vi "GPR Init.vi"(3 "Container State":T10, 4 "Previous State":variant, 5 "Previous Version":T9) -> (2 "Current State":T1={"GPR Graph Info"={"Display Type"=enum."Intensity Plot", "Display Info"={"X Scale"={"X Scale Label"=TRUE, "X Scale Name"="Trace #", "X Scale Visible"=TRUE, "dx"=1.0}, "Y Scale"={"X Scale Label"=TRUE, "X Scale Name"="Time (s)", "X Scale Visible"=TRUE, "dt"=4e-10}, "BackGround Color"=16448250}, "Trace Options"={"Trace Amplitude"=1.0, "Trace Color"=0, "Fill options"=enum."No Fill"}, "Intensity Options"={"Color Scale"=enum."RWB"}}, "Transpose Data"=FALSE, "Run-time Edit"=FALSE, "Clear Request"=FALSE})   [LabVIEW 2009, in "GPR.xctl"]
uses:
  GPR.xctl
  GPR State.ctl
  Controls/GPR Graph Info.ctl
  Controls/Display Types.ctl
  Controls/Display Info.ctl
  Controls/Trace Options.ctl
  Controls/Fill Options.ctl
  Controls/Intensity Options.ctl
  Controls/Color Scales.ctl
  <vilib>/_xctls/Container State.ctl
  <vilib>/_xctls/Version.ctl
  <vilib>/_xctls/XControlSupport.lvlib
panel:
  in  "Default Indicator State":T1={"GPR Graph Info"={"Display Type"=enum."Intensity Plot", "Display Info"={"X Scale"={"X Scale Label"=TRUE, "X Scale Name"="Trace #", "X Scale Visible"=TRUE, "dx"=1.0}, "Y Scale"={"X Scale Label"=TRUE, "X Scale Name"="Time (s)", "X Scale Visible"=TRUE, "dt"=4e-10}, "BackGround Color"=16448250}, "Trace Options"={"Trace Amplitude"=1.0, "Trace Color"=0, "Fill options"=enum."No Fill"}, "Intensity Options"={"Color Scale"=enum."RWB"}}, "Transpose Data"=FALSE, "Run-time Edit"=FALSE, "Clear Request"=FALSE}
  in  "Default Control State":T1={"GPR Graph Info"={"Display Type"=enum."Intensity Plot", "Display Info"={"X Scale"={"X Scale Label"=TRUE, "X Scale Name"="Trace #", "X Scale Visible"=TRUE, "dx"=1.0}, "Y Scale"={"X Scale Label"=TRUE, "X Scale Name"="Time (s)", "X Scale Visible"=TRUE, "dt"=4e-10}, "BackGround Color"=16448250}, "Trace Options"={"Trace Amplitude"=1.0, "Trace Color"=0, "Fill options"=enum."No Fill"}, "Intensity Options"={"Color Scale"=enum."RWB"}}, "Transpose Data"=FALSE, "Run-time Edit"=FALSE, "Clear Request"=FALSE}
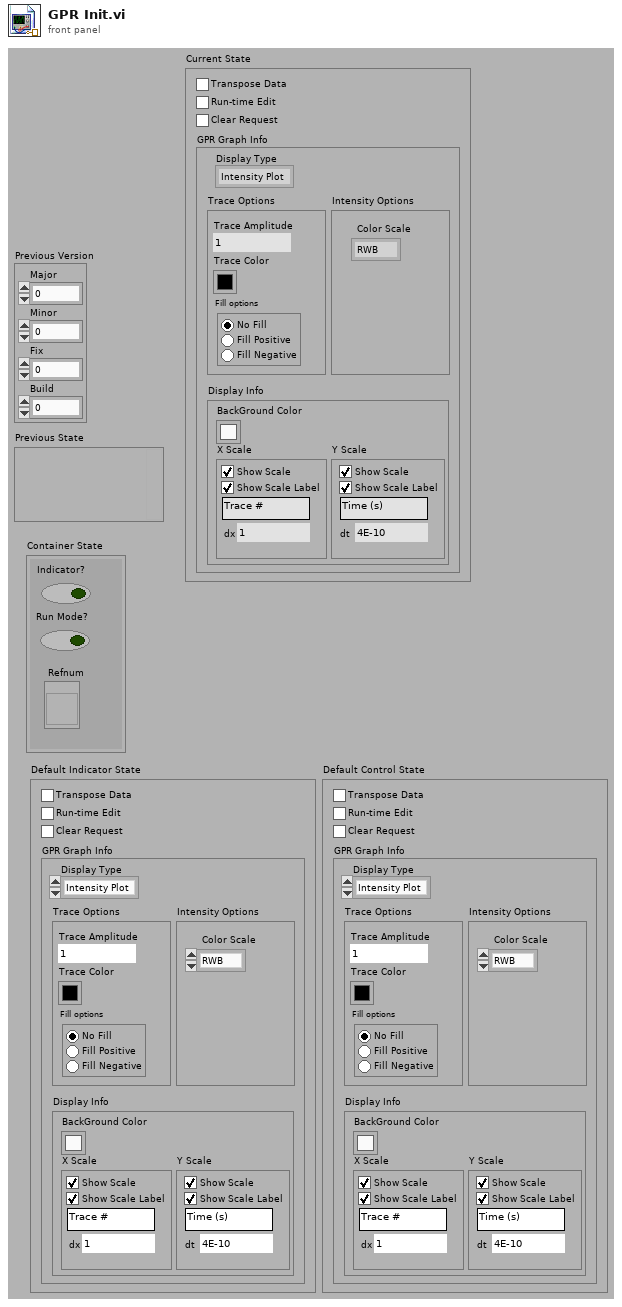
[diagram p1: front panel]
types:
  T1 = typedef "GPR.xctl/GPR State.ctl" = cluster{"GPR Graph Info":T2, "Transpose Data":bool, "Run-time Edit":bool, "Clear Request":bool}
  T2 = typedef "GPR Graph Info.ctl" = cluster{"Display Type":T3, "Display Info":T4, "Trace Options":T5, "Intensity Options":T7}
  T3 = typedef "Display Types.ctl" = enum16{"Intensity Plot", "Wiggle Trace"}
  T4 = typedef "Display Info.ctl" = cluster{"X Scale":cluster{"X Scale Label":bool, "X Scale Name":string, "X Scale Visible":bool, "dx":dbl}, "Y Scale":cluster{"X Scale Label":bool, "X Scale Name":string, "X Scale Visible":bool, "dt":dbl}, "BackGround Color":u32}
  T5 = typedef "Trace Options.ctl" = cluster{"Trace Amplitude":dbl, "Trace Color":u32, "Fill options":T6}
  T6 = typedef "Fill Options.ctl" = enum32{"No Fill", "Fill Positive", "Fill Negative"}
  T7 = typedef "Intensity Options.ctl" = cluster{"Color Scale":T8}
  T8 = typedef "Color Scales.ctl" = enum16{"RGB", "RWB", "BGR", "BWR", "BW", "WB"}
  T9 = typedef "XControlSupport.lvlib/Version.ctl" = cluster{"Major":u16, "Minor":u16, "Fix":u16, "Build":u16}
  T10 = typedef "XControlSupport.lvlib/Container State.ctl" = cluster{"Indicator?":bool, "Run Mode?":bool, " Refnum":refnum<vi>}
  T11 = cluster{"Major":u16, "Minor":u16, "Fix":u16, "Build":u16}
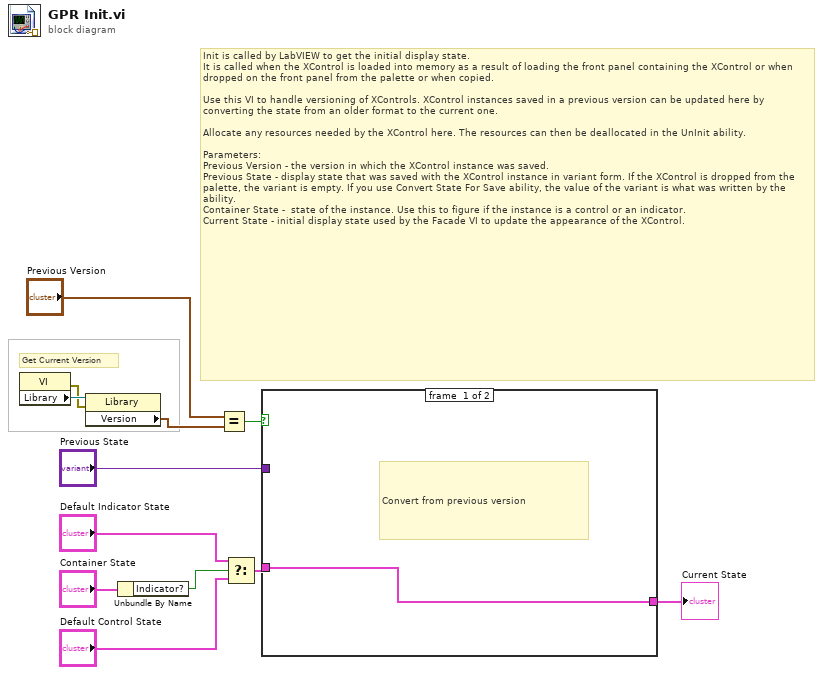
[diagram p0: block diagram]
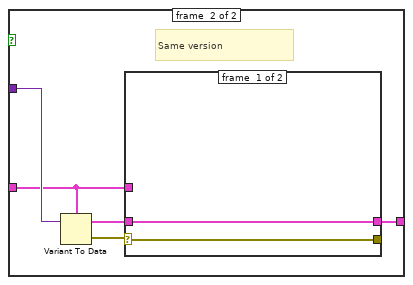
[diagram p2: hidden frame]
diagram:
  # "Get Current Version"
  # "Init is called by LabVIEW to get the initial display state.\nIt is called when the XControl is loaded into memory as a result of loading the front panel containing the XControl or when dropped on the front panel from the palette or when copied.\n\nUse this VI to handle versioning of XControls. XControl instances saved in a previous version can be updated here by converting the state from an older format to the current one.\n\nAllocate any resources needed by the XControl here. The resources can then be deallocated in the UnInit ability.\n\nParameters:\nPrevious Version - the version in which the XControl instance was saved.\nPrevious State - display state that was saved with the XControl instance in variant form. If the XControl is dropped from the palette, the variant is empty. If you use Convert State For Save ability, the value of the variant is what was written by the ability. \nContainer State -  state of the instance. Use this to figure if the instance is a control or an indicator.\nCurrent State - initial display state used by the Facade VI to update the appearance of the XControl."
  n1 = property class="VI"() -> (error out=w2:errorcluster, "Library"=w3:refnum<vi>)  [unwired: 2 in, 1 out]
  n2 = property class="Library"(reference=w3, error in=w2) -> ("Version"=w1:T11)  [unwired: 2 out]
  n3 = Unbundle By Name("Container State") -> ("Indicator?"=w5:bool)
  n4 = Equal?(x="Previous Version", y=w1) -> (x = y?=w11:bool)
  n5 = Select(t="Default Indicator State", s=w5, f="Default Control State") -> (s? t:f=w4:T1)
  n6 = case shown="True" w11 {
    tunnel: "Previous State" -> [_ w18]
    tunnel: [w13 w14] -> w9
    tunnel: w4 -> [w13 w15]
    frame #0 {
      # "Convert from previous version"
    }
    frame #1 {
      # "Same version"
      n7 = Variant To Data(Variant=w18, type=w15) -> (error out=w17:errorcluster, data=w16:T1)  [unwired: 1 in]
      n8 = case shown="Error" w17 {
        selector: w17 -> [w20 w21]
        tunnel: w16 -> [w19 _]
        tunnel: [w19 w22] -> w14
        tunnel: w15 -> [_ w22]
        tunnel: [w20 w21] -> _
        frame #0 {
        }
        frame #1 {
          # "Error converting previously \nsaved state. Use default instead."
        }
      }
    }
  }
  "Current State" <- w9
